vi "Read Waveform Measurement.vi"(6 "Source Channel 2 (2: Channel 2)":u16(ring)=2 items=["Channel 1"=1, "Channel 2"=2, "Channel 3"=3, "Channel 4"=4], 7 "Measurement Function (0: Rise Time)":u16(ring) items=["Rise Time", "Fall Time", "Frequency", "Duty Cycle Negative", "Duty Cycle Positive", "Width Negative", "Width Positive", "Over Shoot", "Pre Shoot", "Period", "Amplitude", "Voltage Average", "Voltage Base", "Voltage Max", "Voltage Min", "Voltage Vpp", "Voltage RMS", "Voltage Top", "Phase Negative", "Phase Positive", "Delay Negative", "Delay Positive"], 8 "error in (no error)":errorcluster, 9 "Maximum Time (10000 ms)":u32=10000, 10 "Source Channel (1: Channel 1)":u16(ring)=1 items=["Channel 1"=1, "Channel 2"=2, "Channel 3"=3, "Channel 4"=4], 11 "VISA resource name":refnum<visa-resource-name>) -> (0 "error out":errorcluster, 2 "Measurement":dbl, 3 "VISA resource name out":refnum<visa-resource-name>)   [LabVIEW 2010, in "Agilent DSO1000 Series.lvlib"]
doc: "Initiates an acquisition on the channels that you enable with the Configure Channel.vi. It then waits for the acquisition to complete, obtains a waveform measurement on the channel you specify, and returns the measurement value. You specify a particular measurement type, such as rise time, frequency, and voltage peak-to-peak. You can call the Fetch Waveform Measurement VI separately for any other waveform measurement that you want to obtain on a specific channel without initiating another acquisition."
uses:
  <instrlib>/Agilent DSO1000 Series/Agilent DSO1000 Series.lvlib
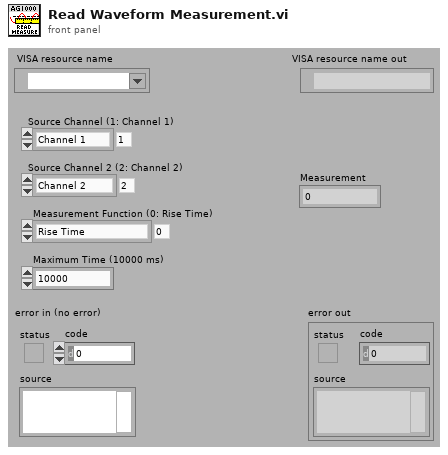
[diagram p1: front panel]
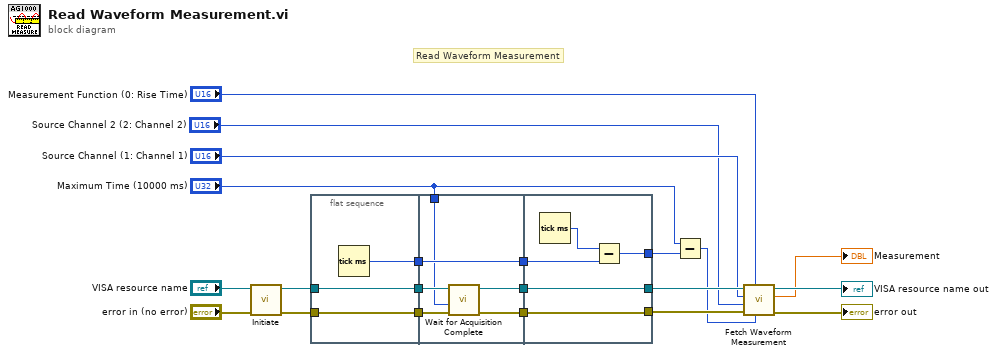
[diagram p0: block diagram]
diagram:
  # "Read Waveform Measurement"
  n1 = call <instrlib>:"Initiate.vi"("error in (no error)"="error in (no error)", "VISA resource name"="VISA resource name") -> ("error out"=w18:errorcluster, "VISA resource name out"=w19:refnum<visa-resource-name>)  [unwired: 8 in]
  n2 = flat-sequence {
    tunnel: w19 -> [w23]
    tunnel: w18 -> [w22]
    tunnel: [w24] -> w17
    tunnel: [w23] -> w15
    tunnel: [w22] -> w14
    tunnel: w17 -> [w30]
    tunnel: [w30] -> w16
    tunnel: w15 -> [w28]
    tunnel: w14 -> [w29]
    tunnel: "Maximum Time (10000 ms)" -> [w27]
    tunnel: [w26] -> w13
    tunnel: [w25] -> w12
    tunnel: w16 -> [w32]
    tunnel: w13 -> [w34]
    tunnel: [w35] -> w8
    tunnel: w12 -> [w35]
    tunnel: [w34] -> w9
    tunnel: [w31] -> w11
    frame #0 {
      n3 = Tick Count (ms)() -> (millisecond timer value=w24:u32)
    }
    frame #1 {
      n4 = call <instrlib>:"Wait for Acquisition Complete.vi"("error in (no error)"=w29, "Maximum Time (10000 ms)"=w27, "VISA resource name"=w28) -> ("error out"=w25:errorcluster, "VISA resource name out"=w26:refnum<visa-resource-name>)  [unwired: 7 in]
    }
    frame #2 {
      n5 = Tick Count (ms)() -> (millisecond timer value=w33:u32)
      n6 = Subtract(x=w33, y=w32) -> (x-y=w31:u32)
    }
  }
  n7 = Subtract(x="Maximum Time (10000 ms)", y=w11) -> (x-y=w5:u32)
  n8 = call <instrlib>:"Fetch Waveform Measurement.vi"("Maximum Time (10000 ms)"=w5, "Measurement Function (0: Rise Time)"="Measurement Function (0: Rise Time)", "error in (no error)"=w8, "Source Channel 2 (2: Channel 2)"="Source Channel 2 (2: Channel 2)", "Source Channel (1: Channel 1)"="Source Channel (1: Channel 1)", "VISA resource name"=w9) -> ("error out"=→"error out":errorcluster, "Measurement"=→"Measurement":dbl, "VISA resource name out"=→"VISA resource name out":refnum<visa-resource-name>)  [unwired: 3 in]
